vi "Get switch channel.vi"(7 "timeout ms (2000)":i32=2000, 8 "error in":errorcluster, 11 "RedPitaya connection in":refnum<k5>) -> (0 "error out":errorcluster, 2 "Channel":i32, 3 "RedPitaya connection out":refnum<k5>)   [LabVIEW 2021]
uses:
  Red_Pitaya_LabVIEW_Driver&Examples/Red_Pitaya/RedPitaya.lvlib
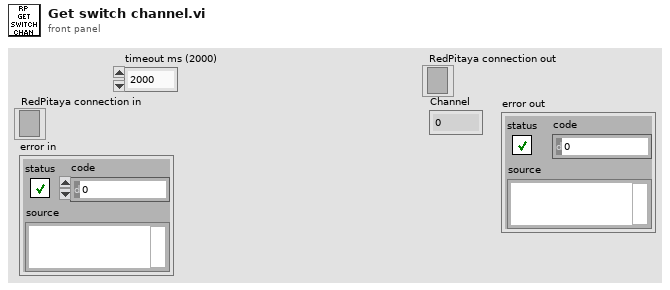
[diagram p1: front panel]
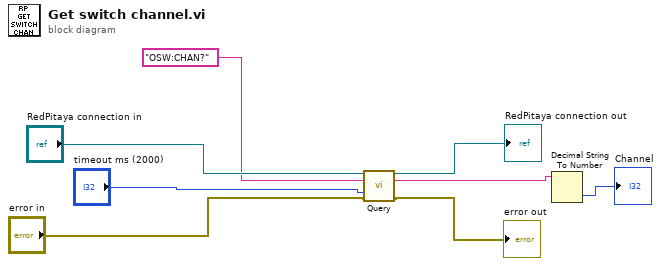
[diagram p0: block diagram]
diagram:
  n1 = call "Query.vi"("RedPitaya connection in"="RedPitaya connection in", "SCPI Query"="OSW:CHAN?" ("format string"), "timeout ms (2000)"="timeout ms (2000)", "error in"="error in") -> ("RedPitaya connection out"=→"RedPitaya connection out":refnum<k5>, "data out"=w2:string, "error out"=→"error out":errorcluster)  [unwired: 9 in]
  n2 = Decimal String To Number(string=w2) -> (number=→"Channel":i32)  [unwired: 2 in, 1 out]
